vi "Signed Array Index.vi"(9 "Array Size":i32, 10 "Array Index in":i32) -> (2 "Array Index out":i32)   [LabVIEW 2021]
doc: "use i[n] as the resulting index, where i is the input index and n is the number of array element, making it a circular array"
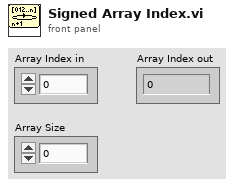
[diagram p1: front panel]
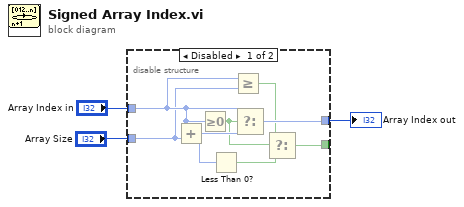
[diagram p0: block diagram]
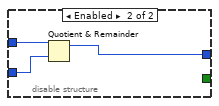
[diagram p2: hidden frame]
diagram:
  n1 = disable-structure shown="Disabled" {
    disable-tunnel: [w11 w12] -> w3
    disable-tunnel: "Array Index in" -> [w10 w14]
    disable-tunnel: "Array Size" -> [w9 w13]
    disable-tunnel: [w4 _] -> _
    frame Disabled {
      n2 = Add(x=w10, y=w9) -> (x+y=w8:i32)
      n3 = Greater Or Equal To 0?(x=w10) -> (x >= 0?=w7:bool)
      n4 = Less Than 0?(x=w8) -> (x < 0?=w5:bool)
      n5 = Greater Or Equal?(x=w10, y=w9) -> (x >= y?=w6:bool)
      n6 = Select(t=w10, s=w7, f=w8) -> (s? t:f=w11:i32)
      n7 = Select(t=w6, s=w7, f=w5) -> (s? t:f=w4:bool)
    }
    frame Enabled {
      n8 = Quotient & Remainder(x=w14, y=w13) -> (x-y*floor(x/y)=w12:i32)  [unwired: 1 out]
    }
  }
  "Array Index out" <- w3
